vi "multipleFramesToOneFrames.vi"(9 "Field Size":T5, 11 "Multiple frames":T1[](array[typedef]) {"robots_blue"."height" format="%+4.3f"; "robots_blue"."pixel_y" format="%+4.3f"; "robots_blue"."pixel_x" format="%+4.3f"; "robots_blue"."orientation" format="%+4.3f"; "robots_blue"."y" format="%+4.3f"; "robots_blue"."confidence" format="%4.3f"; "robots_blue"."x" format="%+4.3f"; "robots_yellow"."height" format="%+4.3f"; "robots_yellow"."pixel_y" format="%+4.3f"; "robots_yellow"."pixel_x" format="%+4.3f"; "robots_yellow"."orientation" format="%+4.3f"; "robots_yellow"."y" format="%+4.3f"; "robots_yellow"."confidence" format="%4.3f"; "robots_yellow"."x" format="%+4.3f"}) -> (3 "Single frame":T1 {"robots_blue"."height" format="%+4.3f"; "robots_blue"."pixel_y" format="%+4.3f"; "robots_blue"."pixel_x" format="%+4.3f"; "robots_blue"."orientation" format="%+4.3f"; "robots_blue"."y" format="%+4.3f"; "robots_blue"."confidence" format="%4.3f"; "robots_blue"."x" format="%+4.3f"; "robots_yellow"."height" format="%+4.3f"; "robots_yellow"."pixel_y" format="%+4.3f"; "robots_yellow"."pixel_x" format="%+4.3f"; "robots_yellow"."orientation" format="%+4.3f"; "robots_yellow"."y" format="%+4.3f"; "robots_yellow"."confidence" format="%4.3f"; "robots_yellow"."x" format="%+4.3f"})   [LabVIEW 2017]
uses:
  SSL Detection Frame.ctl
  SSL Detection Robot.ctl
  <vilib>/Analysis/Matrix/Datatypes/RealMatrix.ctl
  SSL Detection Ball.ctl
  <vilib>/Analysis/Matrix/NI_Matrix.lvlib
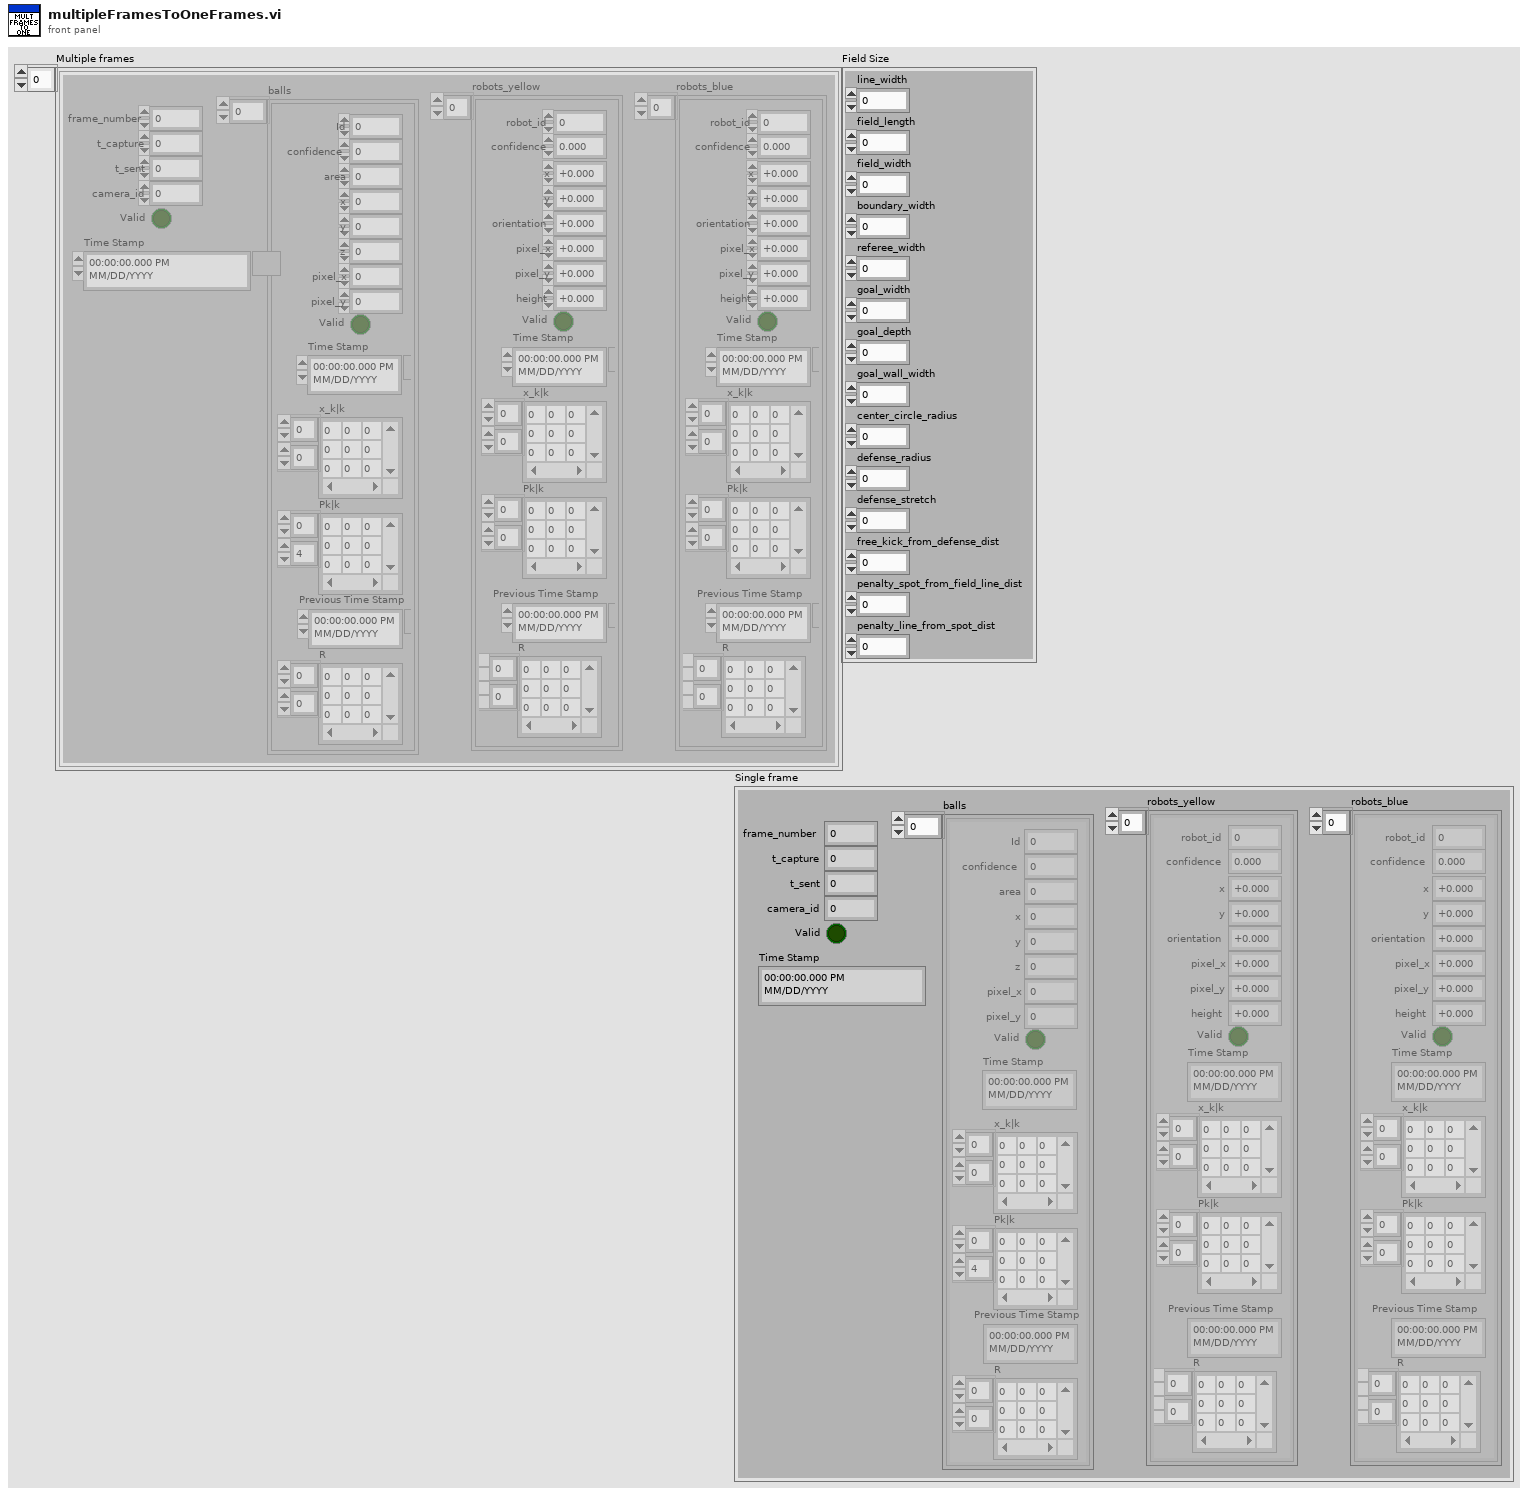
[diagram p1: front panel]
types:
  T1 = typedef "SSL Detection Frame.ctl" = cluster{"frame_number":u32, "t_capture":dbl, "t_sent":dbl, "camera_id":u32, "robots_yellow":T2[], "robots_blue":T2[], "balls":T4[], "Valid":bool, "Time Stamp":timestamp}
  T2 = typedef "SSL Detection Robot.ctl" = cluster{"x":sgl, "robot_id":u32, "confidence":sgl, "y":sgl, "orientation":sgl, "pixel_x":sgl, "pixel_y":sgl, "height":sgl, "Valid":bool, "Time Stamp":timestamp, "x_k|k":T3, "Pk|k":T3, "Previous Time Stamp":timestamp, "R":T3}
  T3 = typedef "NI_Matrix.lvlib/RealMatrix.ctl" = dbl[][]
  T4 = typedef "SSL Detection Ball.ctl" = cluster{"x":sgl, "area":u32, "confidence":sgl, "y":sgl, "z":sgl, "pixel_x":sgl, "pixel_y":sgl, "Valid":bool, "Time Stamp":timestamp, "x_k|k":T3, "Pk|k":T3, "Id":u32, "Previous Time Stamp":timestamp, "R":T3}
  T5 = cluster{"line_width":u32, "field_length":u32, "field_width":u32, "boundary_width":u32, "referee_width":u32, "goal_width":u32, "goal_depth":u32, "goal_wall_width":u32, "center_circle_radius":u32, "defense_radius":u32, "defense_stretch":u32, "free_kick_from_defense_dist":u32, "penalty_spot_from_field_line_dist":u32, "penalty_line_from_spot_dist":u32}
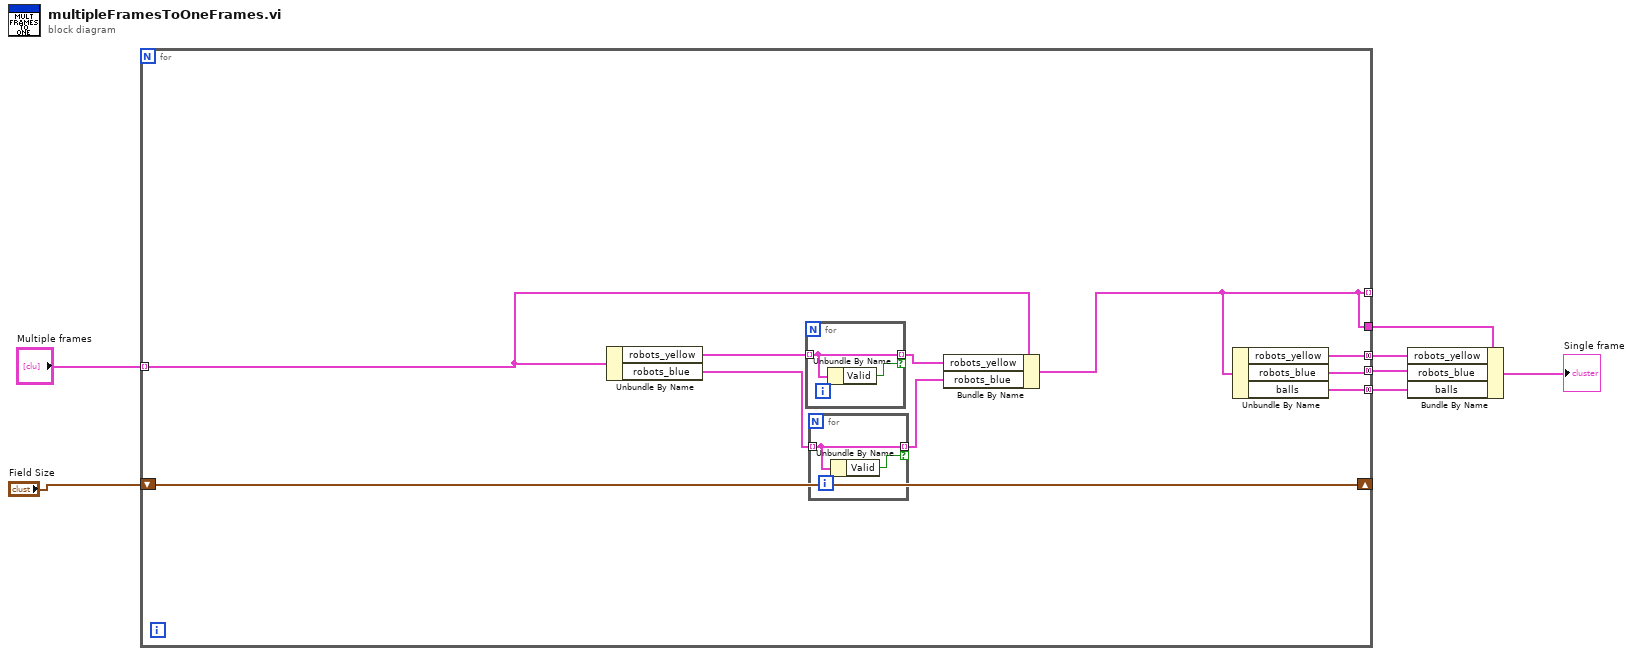
[diagram p0: block diagram]
diagram:
  n1 = for {
    tunnel: [w12] -> _ mode=indexing
    tunnel: "Multiple frames" -> [w16] mode=indexing
    shift-right: [w17] -> _
    shift-left: "Field Size" -> [w17]
    tunnel: [w15] -> w5 mode=concatenating
    tunnel: [w14] -> w4 mode=concatenating
    tunnel: [w13] -> w3 mode=concatenating
    tunnel: [w12] -> w2
    n2 = Unbundle By Name(w16) -> ("robots_yellow"=w11:T2[], "robots_blue"=w9:T2[])
    n3 = for {
      tunnel: w11 -> [w21] mode=indexing
      tunnel: [w21] -> w10 mode=indexing if=w20
      n4 = Unbundle By Name(w21) -> ("Valid"=w20:bool)
    }
    n5 = for {
      tunnel: w9 -> [w19] mode=indexing
      tunnel: [w19] -> w8 mode=indexing if=w18
      n6 = Unbundle By Name(w19) -> ("Valid"=w18:bool)
    }
    n7 = Bundle By Name(cluster=w16, "robots_yellow"=w10, "robots_blue"=w8) -> (w12:T1)
    n8 = Unbundle By Name(w12) -> ("robots_yellow"=w15:T2[], "robots_blue"=w14:T2[], "balls"=w13:T4[])
  }
  n9 = Bundle By Name(cluster=w2, "robots_yellow"=w5, "robots_blue"=w4, "balls"=w3) -> (→"Single frame":T1)
